vi "MotorPositioningVI.vi"(7 "?":bool, 10 "MG17MotorLib.MG17Motor in":refnum<k7>, 11 "Automation Refnum in":refnum<k7>) -> (2 "X Position":sgl, 3 "Angle Position":sgl)   [LabVIEW 2020]
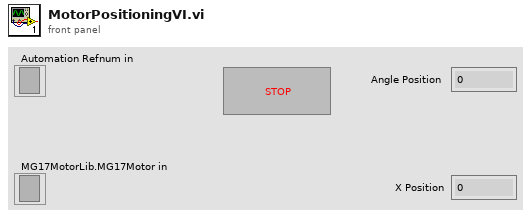
[diagram p1: front panel]
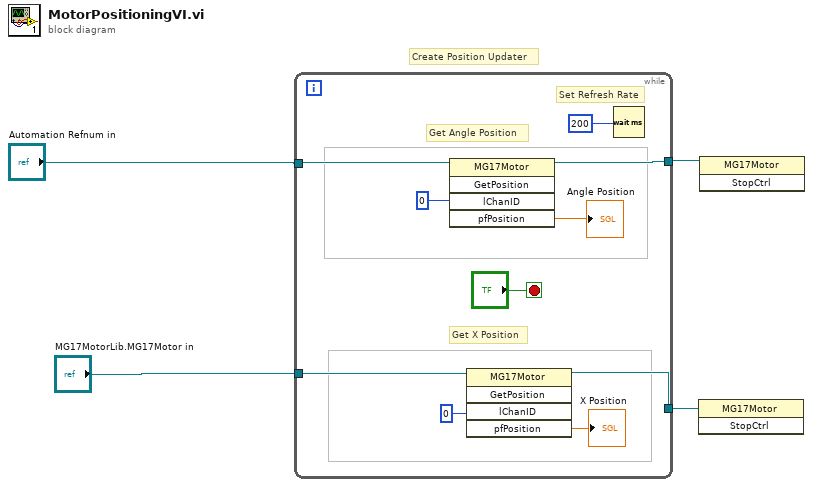
[diagram p0: block diagram]
diagram:
  # "Create Position Updater"
  n1 = while {
    tunnel: [w13] -> w1
    tunnel: "MG17MotorLib.MG17Motor in" -> [w5]
    tunnel: [w7] -> w3
    tunnel: "Automation Refnum in" -> [w6]
    stop <- "?" stop-if-true
    # "Get Angle Position"
    # "Get X Position"
    # "Set Refresh Rate"
    n2 = invoke class="MG17Motor" method="GetPosition"(reference=w6, "lChanID"=0) -> (reference out=w13:refnum<k7>, "pfPosition"=→"Angle Position":sgl)  [unwired: 3 in, 3 out]
    n3 = invoke class="MG17Motor" method="GetPosition"(reference=w5, "lChanID"=0) -> (reference out=w7:refnum<k7>, "pfPosition"=→"X Position":sgl)  [unwired: 3 in, 3 out]
    n4 = Wait (ms)(milliseconds to wait=u32 200 ("millisecond timer value")) -> ()  [unwired: 1 out]
  }
  n5 = invoke class="MG17Motor" method="StopCtrl"(reference=w3) -> ()  [unwired: 2 in, 3 out]
  n6 = invoke class="MG17Motor" method="StopCtrl"(reference=w1) -> ()  [unwired: 2 in, 3 out]
